vi "ArrayIndices(SubVI).vi"(8 "Error In":errorcluster, 10 "Array In":string[](array[string]), 11 "StringsAndValues[]":cluster{"String":string, "Value":string}[](array[cluster])) -> (0 "Error Out":errorcluster, 2 "Array Out":dbl[](array[numeric]))   [LabVIEW 2018]
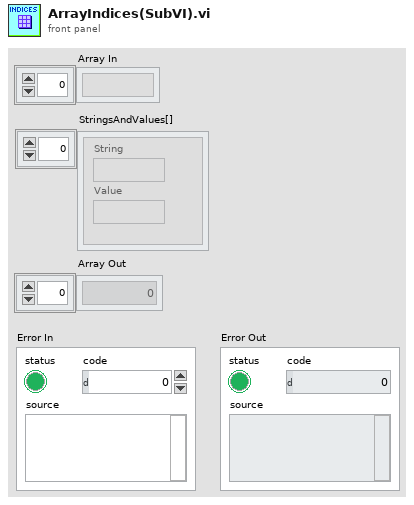
[diagram p1: front panel]
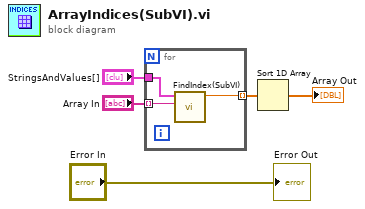
[diagram p0: block diagram]
diagram:
  n1 = for {
    tunnel: "Array In" -> [w8] mode=indexing
    tunnel: "StringsAndValues[]" -> [w7]
    tunnel: [w6] -> w2 mode=indexing
    n2 = call "FindIndex(SubVI).vi"("Name"=w8, "Strings And Values[]"=w7) -> ("Index"=w6:dbl)  [unwired: 8 in, 1 out]
  }
  n3 = Sort 1D Array(array=w2) -> (sorted array=→"Array Out":dbl[])
  "Error Out" <- "Error In"
